vi "Rapid Read_2Ch.vi"(0 "NI Card 3":refnum<k15>, 2 "Pause?":bool, 5 "Motion Board ID":T1=1 min=1 max=32 step=1, 9 "rf points per line":i32, 11 "error in":errorcluster, 12 "lines per plane":i32, 13 "queue out":refnum<queue>) -> (1 "gain":dbl, 6 "Reverse?":bool, 10 "Dig Word Size":u16, 15 "error out":errorcluster)   [LabVIEW 2022 SP3]
uses:
  Motion Controllers/-MotionRoutines/MotionGlobals.vi
  <instrlib>/niScope/Acquire/Fetch/niScope Multi Fetch Binary 8.vi
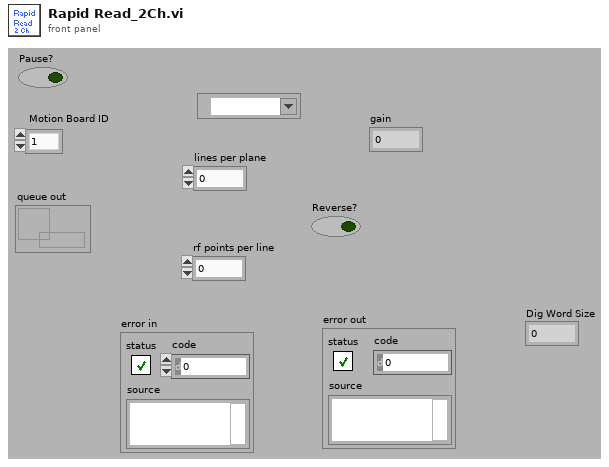
[diagram p1: front panel]
types:
  T1 = typedef "Board Id" = u8
  T2 = typedef "Var" = u8
  T3 = cluster{"actualSamples":i32, "absoluteInitialX":dbl, "relativeInitialX":dbl, "xIncrement":dbl, "offset":dbl, "gain":dbl, "reserved1":dbl, "reserved2":dbl}[]
  T4 = cluster{"actualSamples":i32, "absoluteInitialX":dbl, "relativeInitialX":dbl, "xIncrement":dbl, "offset":dbl, "gain":dbl, "reserved1":dbl, "reserved2":dbl}
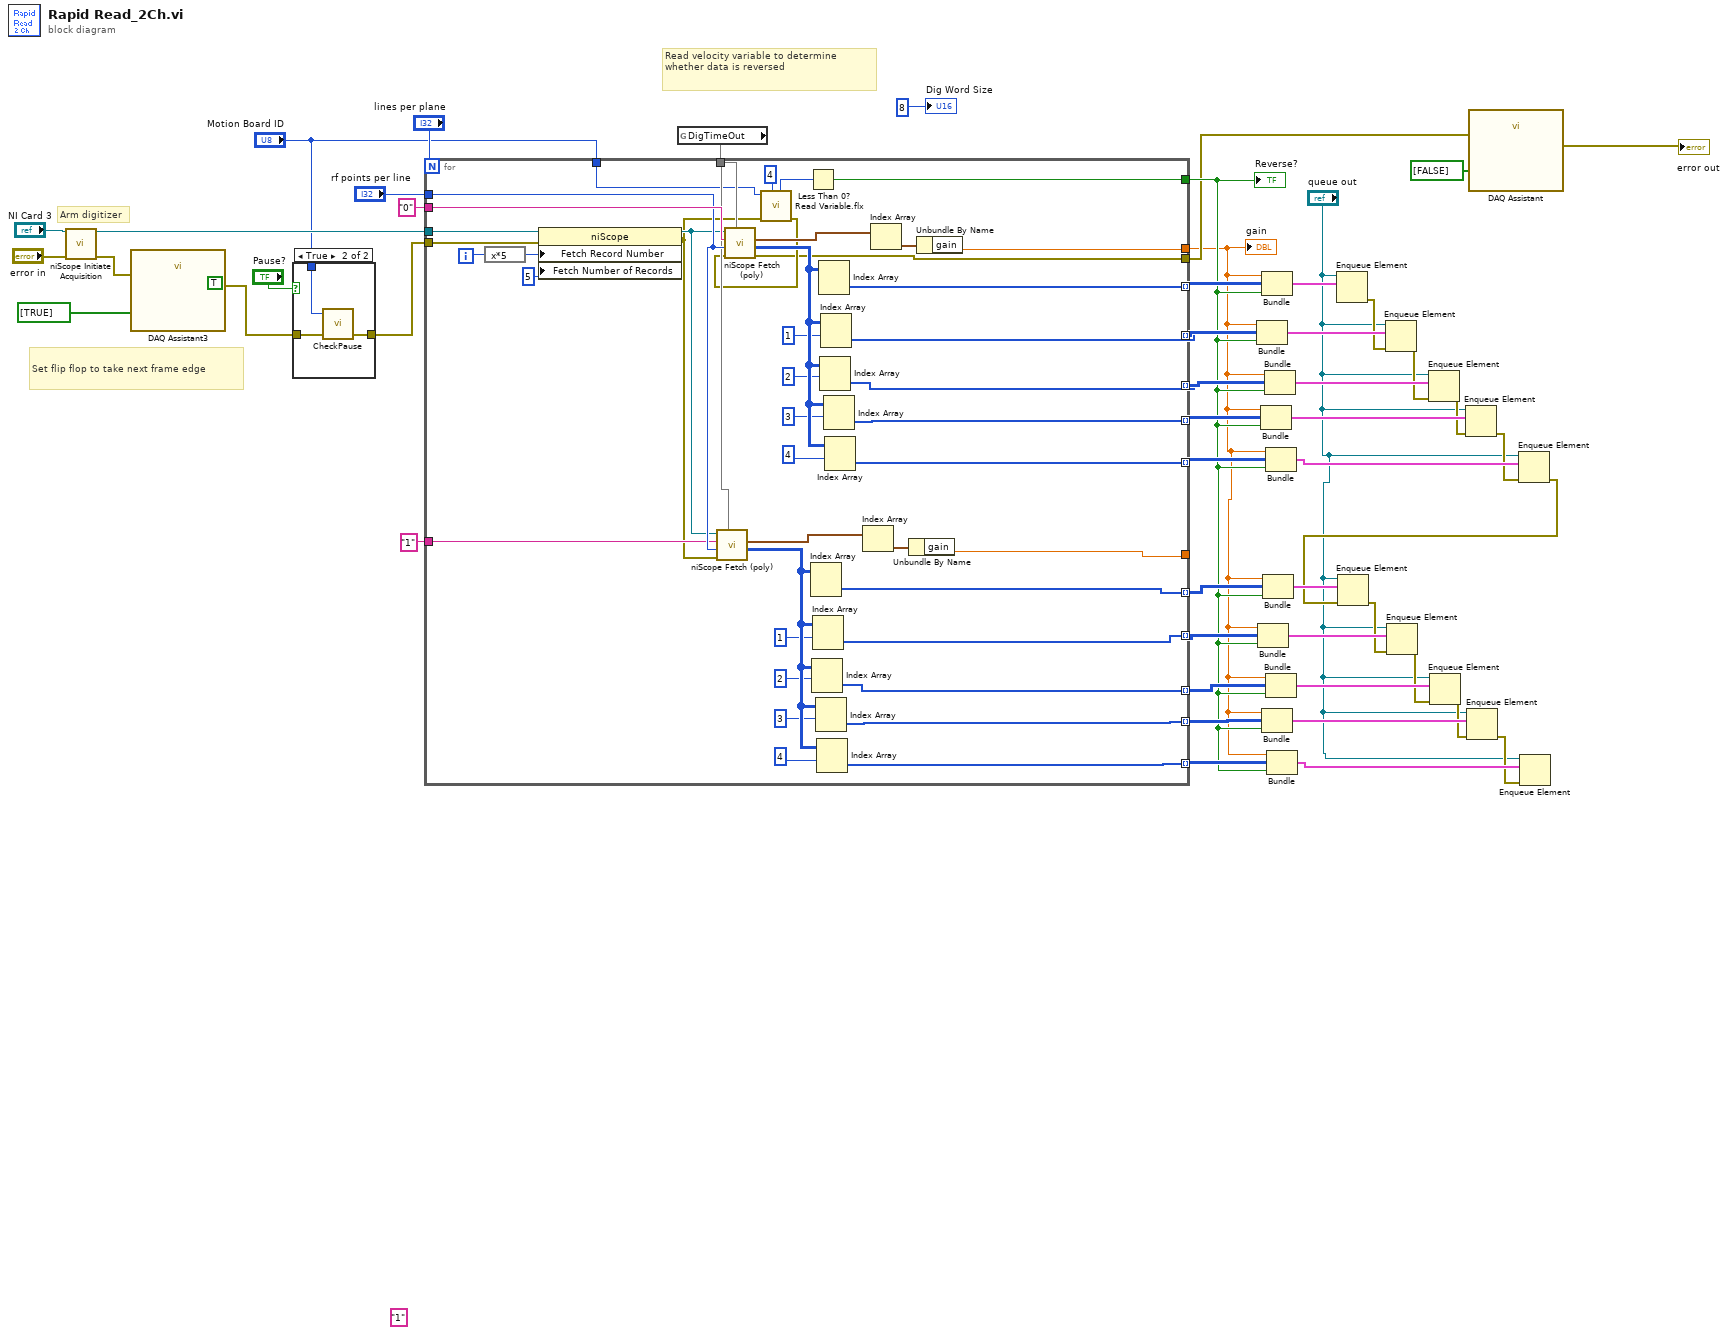
[diagram p0: block diagram]
diagram:
  (unwired) "1" ("Channel")
  (unwired) TRUE ("stop (T)")
  # "Set flip flop to take next frame edge"
  # "Arm digitizer"
  # "Read velocity variable to determine whether data is reversed"
  n1 = call <instrlib>:"niScope Initiate Acquisition.vi"("instrument handle"="NI Card 3", "error in"="error in") -> ("instrument handle out"=w5:refnum<k15>, "error out"=w46:errorcluster)  [unwired: 1 in, 11 out]
  n2 = call "DAQ Assistant3"("data"=bool[] [TRUE], "error in"=w46) -> ("error out"=w4:errorcluster)  [unwired: 2 in, 15 out]
  n3 = case shown="True" "Pause?" {
    tunnel: w4 -> [w51 w54]
    tunnel: [w51 w53] -> w3
    tunnel: "Motion Board ID" -> [_ w52]
    frame False {
    }
    frame True {
      n4 = call "CheckPause.vi"("error in"=w54, "Motion Board ID"=w52) -> ("error out"=w53:errorcluster)  [unwired: 3 in]
    }
  }
  n5 = global read "MotionGlobals.vi" "DigTimeOut"() -> (w20)
  n6 = for {
    N: "lines per plane" -> [_]
    tunnel: "rf points per line" -> [w72]
    tunnel: w20 -> [w70]
    tunnel: w5 -> [w97]
    tunnel: "0" ("Channel") -> [w92]
    tunnel: [w86] -> w35 mode=indexing
    tunnel: [w85] -> w34 mode=indexing
    tunnel: [w84] -> w33 mode=indexing
    tunnel: [w83] -> w32 mode=indexing
    tunnel: [w82] -> w31 mode=indexing
    tunnel: [w80] -> w7
    tunnel: [w69] -> w17 mode=indexing
    tunnel: [w68] -> w16 mode=indexing
    tunnel: [w67] -> w15 mode=indexing
    tunnel: [w66] -> w14 mode=indexing
    tunnel: [w65] -> w13 mode=indexing
    tunnel: [w64] -> _
    tunnel: "1" ("Channel") -> [w63]
    tunnel: w3 -> [w62]
    tunnel: [w57] -> w10
    tunnel: [w56] -> w9
    tunnel: "Motion Board ID" -> [w55]
    i -> [w93]
    n7 = expression code="x*5"(w93) -> (w94:i32)
    n8 = property class="niScope"(reference=w97, error in=w62, "Fetch Record Number"=w94, "Fetch Number of Records"=5) -> (reference out=w71:refnum<k15>, error out=w59:errorcluster)
    n9 = call-poly <instrlib>:"niScope Fetch (poly).vi"("timeout"=w70, "error in"=w59, "numSamples"=w72, "channels"=w63, "instrument handle"=w71) -> ("wfm"=w78:i8[][], "wfm info"=w79:T3)  [unwired: 5 out]
    n10 = call <vilib>:"Read Variable.flx"("Var"=T2 4, "error in (no error)"=w59, "Board ID"=w55) -> ("error out"=w58:errorcluster, "Output"=w60:i32)  [unwired: 1 in, 4 out]
    n11 = call-poly <instrlib>:"niScope Fetch (poly).vi"("timeout"=w70, "error in"=w58, "numSamples"=w72, "channels"=w92, "instrument handle"=w71) -> ("error out"=w56:errorcluster, "wfm"=w91:i8[][], "wfm info"=w96:T3)  [unwired: 4 out]
    n12 = Less Than 0?(x=w60) -> (x < 0?=w57:bool)
    n13 = Index Array(array=w78) -> (element=w69:i8[])  [unwired: 2 in]
    n14 = Index Array(array=w78, index (row)=2) -> (element=w67:i8[])  [unwired: 1 in]
    n15 = Index Array(array=w78, index (row)=1) -> (element=w68:i8[])  [unwired: 1 in]
    n16 = Index Array(array=w78, index (row)=3) -> (element=w66:i8[])  [unwired: 1 in]
    n17 = Index Array(array=w78, index (row)=4) -> (element=w65:i8[])  [unwired: 1 in]
    n18 = Index Array(array=w91) -> (element=w86:i8[])  [unwired: 2 in]
    n19 = Index Array(array=w91, index (row)=2) -> (element=w84:i8[])  [unwired: 1 in]
    n20 = Index Array(array=w91, index (row)=1) -> (element=w85:i8[])  [unwired: 1 in]
    n21 = Index Array(array=w91, index (row)=3) -> (element=w83:i8[])  [unwired: 1 in]
    n22 = Index Array(array=w91, index (row)=4) -> (element=w82:i8[])  [unwired: 1 in]
    n23 = Index Array(array=w79) -> (element=w73:T4)  [unwired: 1 in]
    n24 = Index Array(array=w96) -> (element=w81:T4)  [unwired: 1 in]
    n25 = Unbundle By Name(w73) -> ("gain"=w64:dbl)
    n26 = Unbundle By Name(w81) -> ("gain"=w80:dbl)
  }
  "Reverse?" <- w10
  "gain" <- w7
  n27 = Bundle("gain"=w7, "wfm"=w34, w10) -> (w43:cluster{"gain":dbl, "wfm":i8[][], bool})  [unwired: 1 in]
  n28 = Bundle("gain"=w7, "wfm"=w16, w10) -> (w29:cluster{"gain":dbl, "wfm":i8[][], bool})  [unwired: 1 in]
  n29 = Bundle("gain"=w7, "wfm"=w32, w10) -> (w41:cluster{"gain":dbl, "wfm":i8[][], bool})  [unwired: 1 in]
  n30 = Bundle("gain"=w7, "wfm"=w35, w10) -> (w44:cluster{"gain":dbl, "wfm":i8[][], bool})  [unwired: 1 in]
  n31 = Bundle("gain"=w7, "wfm"=w14, w10) -> (w27:cluster{"gain":dbl, "wfm":i8[][], bool})  [unwired: 1 in]
  n32 = Bundle("gain"=w7, "wfm"=w17, w10) -> (w30:cluster{"gain":dbl, "wfm":i8[][], bool})  [unwired: 1 in]
  n33 = Bundle("gain"=w7, "wfm"=w33, w10) -> (w42:cluster{"gain":dbl, "wfm":i8[][], bool})  [unwired: 1 in]
  n34 = Bundle("gain"=w7, "wfm"=w31, w10) -> (w40:cluster{"gain":dbl, "wfm":i8[][], bool})  [unwired: 1 in]
  n35 = Bundle("gain"=w7, "wfm"=w15, w10) -> (w28:cluster{"gain":dbl, "wfm":i8[][], bool})  [unwired: 1 in]
  n36 = Bundle("gain"=w7, "wfm"=w13, w10) -> (w26:cluster{"gain":dbl, "wfm":i8[][], bool})  [unwired: 1 in]
  n37 = Enqueue Element(queue="queue out", element=w44) -> (error out=w39:errorcluster)  [unwired: 2 in, 2 out]
  n38 = Enqueue Element(queue="queue out", element=w43, error in (no error)=w39) -> (error out=w38:errorcluster)  [unwired: 1 in, 2 out]
  n39 = Enqueue Element(queue="queue out", element=w42, error in (no error)=w38) -> (error out=w37:errorcluster)  [unwired: 1 in, 2 out]
  n40 = Enqueue Element(queue="queue out", element=w41, error in (no error)=w37) -> (error out=w36:errorcluster)  [unwired: 1 in, 2 out]
  n41 = call "DAQ Assistant"("data"=bool[] [FALSE], "error in"=w9) -> ("error out"=→"error out":errorcluster)  [unwired: 2 in, 15 out]
  n42 = Enqueue Element(queue="queue out", element=w40, error in (no error)=w36) -> (error out=w21:errorcluster)  [unwired: 1 in, 2 out]
  n43 = Enqueue Element(queue="queue out", element=w30, error in (no error)=w21) -> (error out=w25:errorcluster)  [unwired: 1 in, 2 out]
  n44 = Enqueue Element(queue="queue out", element=w29, error in (no error)=w25) -> (error out=w24:errorcluster)  [unwired: 1 in, 2 out]
  n45 = Enqueue Element(queue="queue out", element=w28, error in (no error)=w24) -> (error out=w23:errorcluster)  [unwired: 1 in, 2 out]
  n46 = Enqueue Element(queue="queue out", element=w27, error in (no error)=w23) -> (error out=w22:errorcluster)  [unwired: 1 in, 2 out]
  n47 = Enqueue Element(queue="queue out", element=w26, error in (no error)=w22) -> ()  [unwired: 1 in, 3 out]
  "Dig Word Size" <- 8
